vi "act-0019-2-cor.vi"() -> ()   [LabVIEW 2010]
uses:
  support/lv_07.lvlib
panel:
  out "error out":errorcluster caption="err out"
  in  "err in":errorcluster
  out "Qe":dbl
  in  "Pu":dbl
  in  "Qa":dbl
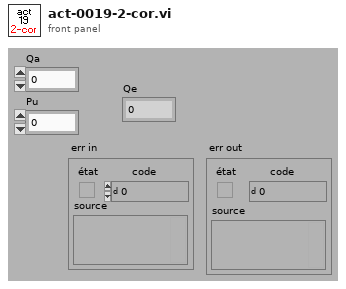
[diagram p1: front panel]
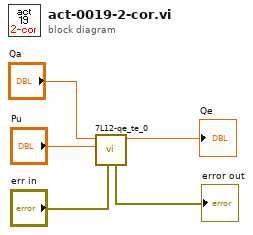
[diagram p0: block diagram]
diagram:
  n1 = call "7L12-qe_te_0.vi"("err in"="err in", "Pu"="Pu", "Qa"="Qa") -> ("Qe"=→"Qe":dbl, "error out"=→"error out":errorcluster)  [unwired: 6 in, 1 out]
